vi "Get Timing.vi"(8 "error in (no error)":errorcluster, 11 "Red Pitaya Digitizer in":refnum<class "Red Pitaya Digitizer.lvclass">) -> (0 "error out":errorcluster, 1 "Decimation":i32=1, 2 "Rate":dbl=125000000.0 format="%#_6pHz", 3 "Red Pitaya Digitizer out":refnum<class "Red Pitaya Digitizer.lvclass">)   [LabVIEW 2024, in "Red Pitaya Digitizer.lvclass"]
uses:
  Red Pitaya Digitizer.lvclass
  Red Pitaya Digitizer.lvclass/Red Pitaya Digitizer.ctl
panel:
  out "In Range?":bool
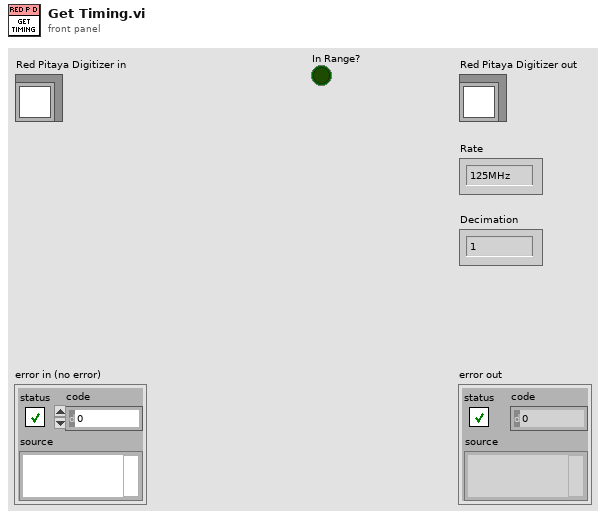
[diagram p1: front panel]
types:
  T1 = typedef "Pusle Driver Configuration.ctl" = cluster{"Post-trigger delay":dbl, "Post-trigger duration":dbl, "Rate":dbl, "Ranges":dbl[], "Re-name channels":string[], "Active channels":string, "External clock":bool}
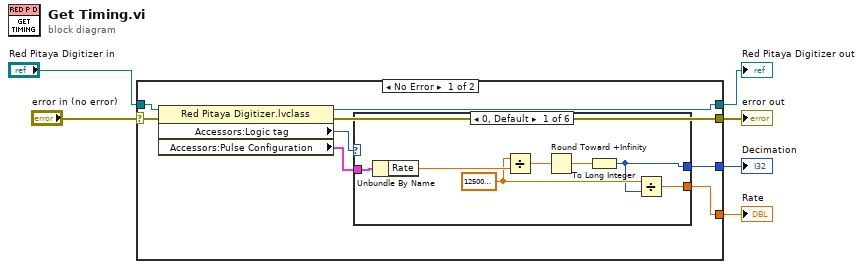
[diagram p0: block diagram]
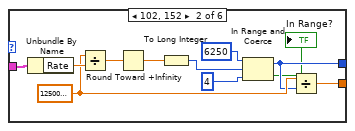
[diagram p2: hidden frame]
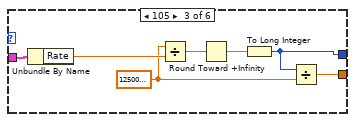
[diagram p3: hidden frame]
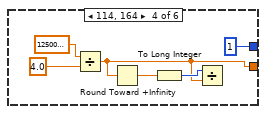
[diagram p4: hidden frame]
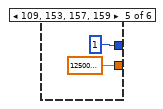
[diagram p5: hidden frame]
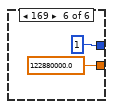
[diagram p6: hidden frame]
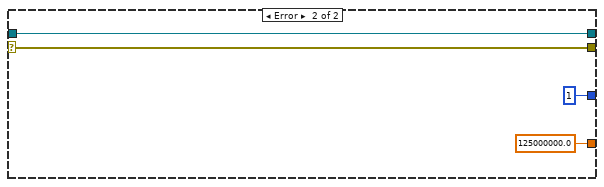
[diagram p7: hidden frame]
diagram:
  n1 = case shown="No Error" "error in (no error)" {
    selector: "error in (no error)" -> [w14 w53]
    tunnel: [w13 w53] -> w5
    tunnel: [w11 w52] -> w3
    tunnel: "Red Pitaya Digitizer in" -> [w12 w52]
    tunnel: [w9 1] -> w2
    tunnel: [w8 125000000.0 ("y")] -> w1
    frame No Error {
      n2 = property class="Red Pitaya Digitizer.lvclass"(reference=w12, error in=w14) -> (reference out=w11:refnum<class "Red Pitaya Digitizer.lvclass">, error out=w13:errorcluster, "Accessors:Logic tag"=w10:u16, "Accessors:Pulse Configuration"=w7:T1)
      n3 = case shown="0, Default" w10 {
        tunnel: w7 -> [w21 w32 w39 _ _ _]
        tunnel: [w15 w23 w35 1 1 1] -> w9
        tunnel: [w17 w28 w33 w41 125000000.0 ("y") 122880000.0 ("y")] -> w8
        frame 0, Default {
          w16 = 125000000.0 ("y")
          n4 = Unbundle By Name(w21) -> ("Rate"=w18:dbl)
          n5 = Divide(x=w16, y=w18) -> (x/y=w19:dbl)
          n6 = Round Toward +Infinity(x=w19) -> (ceil(x): smallest int >= x=w20:dbl)
          n7 = To Long Integer(number=w20) -> (32bit integer=w15:i32)
          n8 = Divide(x=w16, y=w15) -> (x/y=w17:dbl)
        }
        frame 102, 152 {
          w27 = 125000000.0 ("y")
          n9 = Unbundle By Name(w32) -> ("Rate"=w29:dbl)
          n10 = Divide(x=w27, y=w29) -> (x/y=w30:dbl)
          n11 = Round Toward +Infinity(x=w30) -> (ceil(x): smallest int >= x=w31:dbl)
          n12 = To Long Integer(number=w31) -> (32bit integer=w24:i32)
          n13 = In Range and Coerce(upper limit=6250, x=w24, lower limit=4) -> (coerced(x)=w23:i32, In Range?=→"In Range?":bool)
          n14 = Divide(x=w27, y=w23) -> (x/y=w28:dbl)
        }
        frame 105 {
          w34 = 125000000.0 ("y")
          n15 = Unbundle By Name(w39) -> ("Rate"=w36:dbl)
          n16 = Divide(x=w34, y=w36) -> (x/y=w37:dbl)
          n17 = Round Toward +Infinity(x=w37) -> (ceil(x): smallest int >= x=w38:dbl)
          n18 = To Long Integer(number=w38) -> (32bit integer=w35:i32)
          n19 = Divide(x=w35, y=w34) -> (x/y=w33:dbl)
        }
        frame 114, 164 {
          n20 = Divide(x=125000000.0 ("y"), y=4.0) -> (x/y=w41:dbl)
          n21 = Round Toward +Infinity(x=w41) -> (ceil(x): smallest int >= x=w45:dbl)
          n22 = To Long Integer(number=w45) -> (32bit integer=w44:i32)
          n23 = Divide(x=w44, y=w41) -> ()  [unwired: 1 out]
        }
        frame 109, 153, 157, 159 {
        }
        frame 169 {
        }
      }
    }
    frame Error {
    }
  }
  "error out" <- w5
  "Red Pitaya Digitizer out" <- w3
  "Decimation" <- w2
  "Rate" <- w1
